vi "Control Camera Properties.vi"(8 "error in":errorcluster, 10 "Control Camera Properties":T2, 11 "Session In":T1) -> (0 "error out 2":errorcluster, 3 "Session Out 2":T1)   [LabVIEW 2014]
uses:
  <vilib>/userdefined/High Color/IMAQdx.ctl
  <resource>/objmgr/imaqdx.rc
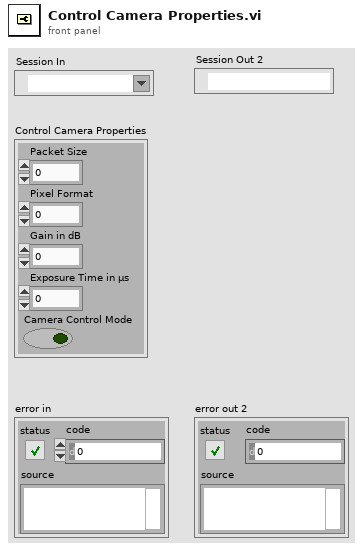
[diagram p1: front panel]
types:
  T1 = typedef "IMAQdx.ctl" = refnum<k21>
  T2 = cluster{"Packet Size":u32, "Pixel Format":u32, "Gain in dB":dbl, "Exposure Time in µs":u32, "Camera Control Mode":bool}
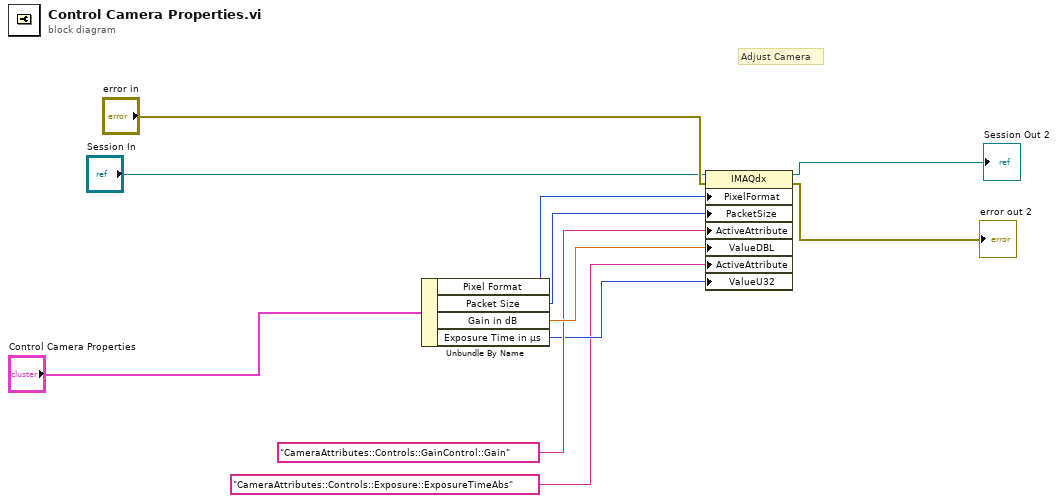
[diagram p0: block diagram]
diagram:
  # "Adjust Camera"
  n1 = Unbundle By Name("Control Camera Properties") -> ("Pixel Format"=w8:u32, "Packet Size"=w7:u32, "Gain in dB"=w6:dbl, "Exposure Time in µs"=w4:u32)
  n2 = property class="IMAQdx"(reference="Session In", error in="error in", "PixelFormat"=w8, "PacketSize"=w7, "ActiveAttribute"="CameraAttributes::Controls::GainControl::Gain", "ValueDBL"=w6, "ActiveAttribute"="CameraAttributes::Controls::Exposure::ExposureTimeAbs", "ValueU32"=w4) -> (reference out=→"Session Out 2":T1, error out=→"error out 2":errorcluster)
